vi "rad_Add Name and Version to Path.vi"(8 "File Extension":string=".lvbitx", 9 "Version":string, 10 "Name":string, 11 "Starting Path":path) -> (2 "filename without extension":string, 3 "New Path":path)   [LabVIEW 2020]
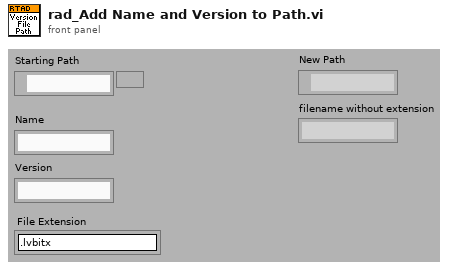
[diagram p1: front panel]
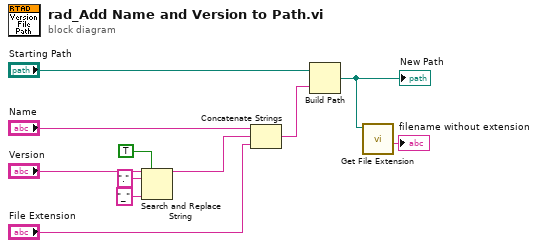
[diagram p0: block diagram]
diagram:
  n1 = Search and Replace String(replace all?=TRUE ("replace all? (F)"), input string="Version", search string=".", replace string="_" ("replace string (\"\")")) -> (result string=w6:string)  [unwired: 4 in, 3 out]
  n2 = Concatenate Strings("Name", w6, "File Extension") -> (w4:string)
  n3 = Build Path(base path="Starting Path", name or relative path=w4) -> (appended path=w2:path)
  "New Path" <- w2
  n4 = call <vilib>:"Get File Extension.vi"("file"=w2) -> ("filename without extension"=→"filename without extension":string)  [unwired: 6 in, 4 out]
